vi "Controller Configure Ethercat.vi"(8 "error in (no error)":errorcluster) -> (0 "error out":errorcluster)   [LabVIEW 2011, in "Controller VIs.lvlib"]
doc: "Configure masters and slaves of Aqcuisition and Actuation EtherCAT networks."
uses:
  Controller VIs.lvlib
  Program Files (x86)/National Instruments/LabVIEW 2011/resource/objmgr/IndComECAT.rc
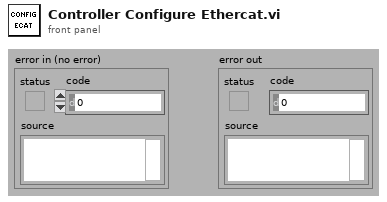
[diagram p1: front panel]
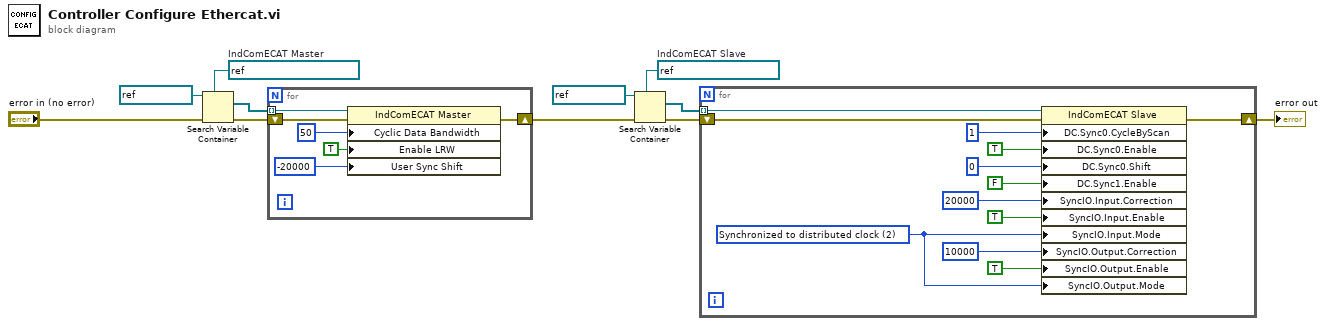
[diagram p0: block diagram]
diagram:
  w7 = refnum<k21> refnum  # IndComECAT Slave
  w2 = refnum<k21> refnum  # IndComECAT Master
  n1 = Search Variable Container(7:w2, 8:"error in (no error)", 11:refnum<k21> "ni.var.io:" ("Master Constant")) -> (0:w4:errorcluster, 2:w3:refnum<k21>[])  [unwired: 3 in, 1 out]
  n2 = for {
    tunnel: w3 -> [w16] mode=indexing
    shift-right: [w15] -> w9
    shift-left: w4 -> [w17]
    n3 = property class="IndComECAT Master"(reference=w16, error in=w17, "Cyclic Data Bandwidth"=u32 50, "Enable LRW"=TRUE, "User Sync Shift"=-20000) -> (error out=w15:errorcluster)  [unwired: 1 out]
  }
  n4 = Search Variable Container(7:w7, 8:w9, 11:refnum<k21> "ni.var.io:" ("Master Constant")) -> (0:w5:errorcluster, 2:w6:refnum<k21>[])  [unwired: 3 in, 1 out]
  n5 = for {
    tunnel: w6 -> [w19] mode=indexing
    shift-right: [w20] -> w11
    shift-left: w5 -> [w18]
    w28 = u32 2 items=["Unsynchronized", "Synchronized to EtherCAT frame", "Synchronized to distributed clock"] ("SyncIO:Output:Mode")
    n6 = property class="IndComECAT Slave"(reference=w19, error in=w18, "DC.Sync0.CycleByScan"=u32 1 ("DC:Sync0:CycleByScan"), "DC.Sync0.Enable"=TRUE ("DC:Sync0:Enable"), "DC.Sync0.Shift"=u32 0 ("DC:Sync0:Shift"), "DC.Sync1.Enable"=FALSE ("DC:Sync1:Enable"), "SyncIO.Input.Correction"=20000 ("User Sync Shift"), "SyncIO.Input.Enable"=TRUE ("SyncIO:Input:Enable"), "SyncIO.Input.Mode"=w28, "SyncIO.Output.Correction"=10000 ("SyncIO:Output:Correction"), "SyncIO.Output.Enable"=TRUE ("SyncIO:Output:Enable"), "SyncIO.Output.Mode"=w28) -> (error out=w20:errorcluster)  [unwired: 1 out]
  }
  "error out" <- w11
